vi "Voltage_overflow_checker.vi"() -> ()   [LabVIEW 2017]
uses:
  Globals/Meas_global.vi
panel:
  out "Over/Under string":string
  out "Extra Comments":string
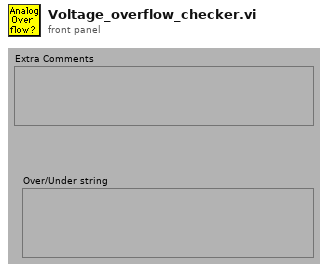
[diagram p1: front panel]
types:
  T1 = typedef "Analysis_info_cluster.ctl" = cluster{"Colour":u32, "Inst type":T2, "Inst name":string, "Symbol":string, "Code name":string, "Extra Info":string, "Inst Array":T3, "Extra Titles":string[], "Extra Values":string[], "U":dbl, "u^2":dbl, "u^3":dbl, "u^4":dbl, "Skew_u":dbl, "Kurt_u":dbl, "Sd Error in Mean":dbl, "% u'/U":dbl, "X":dbl, "Y":dbl, "Z":dbl, "Timescale integral Estimate":dbl, "Sd Error in Variance":dbl, "Calib File":path, "Calib Constants":dbl[], "Output Position":bool, "Full Stats":bool, "Av Sampling Rate":dbl, "Av No of Samples":dbl, "Total Meas Time (s)":dbl, "ADAM Ch Name":string, "Max value":dbl, "Min value":dbl, "Req Sample Rate Hz":dbl, "Sync Delay Time (s)":dbl, "Ch No":i16, "Device":string, "Use Latest Calib":bool, "Port":string, "Metadata Ch Names":string[], "Metadata Ch Values":string[]}
  T2 = typedef "Inst_type.ctl" = enum16{"Propeller anemometer", "Raw voltage", "Pressure Transducer", "Pitot-static tube", "Preston tube", "Hot wire", "Cross wire 1", "Cross wire 2", "Generic Linear", "Generic Polynomial", "Generic BackPoly", "Fast FID", "Thermocouple", "Cold wire", "Pulsed Wire", "LDA Vel", "LDA Tran time", "LDA Arr time", "Microphone"}
  T3 = typedef "Instrument_Array.ctl" = enum16{"PWA", "LDA", "Analogue"}
  T4 = typedef "Time_Trace_Cluster.ctl" = cluster{"Weighting":dbl[], "Time (s)":dbl[], "Voltage":dbl[], "Eng Values":dbl[]}
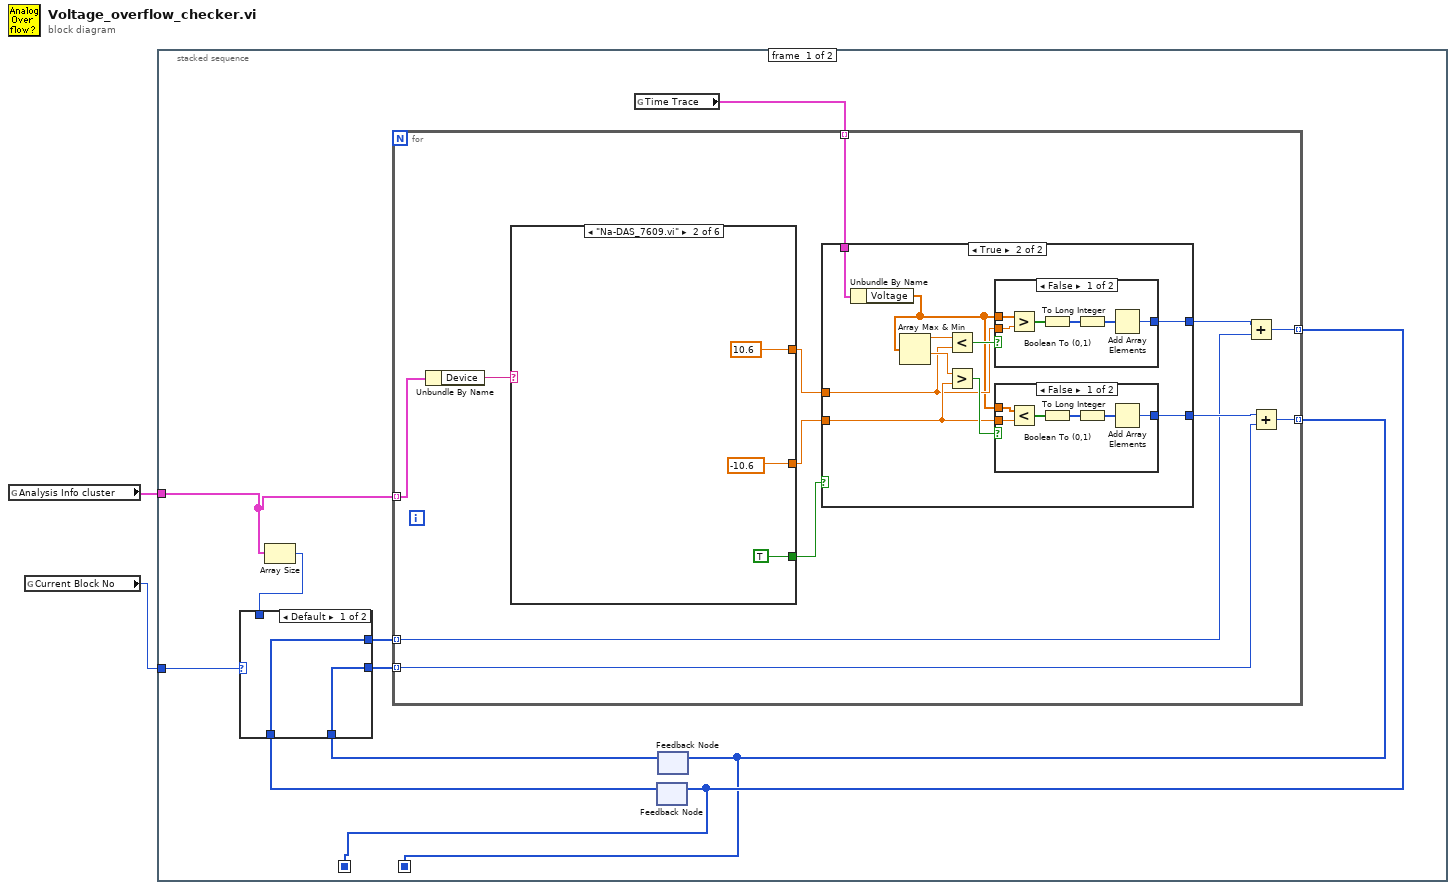
[diagram p0: block diagram]
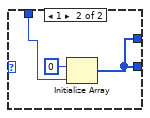
[diagram p2: hidden frame]
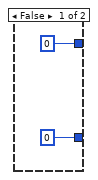
[diagram p3: hidden frame]
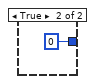
[diagram p4: hidden frame]
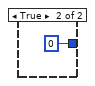
[diagram p5: hidden frame]
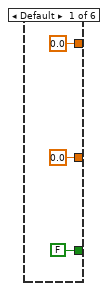
[diagram p6: hidden frame]
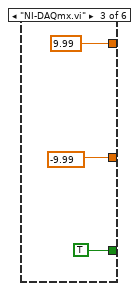
[diagram p7: hidden frame]
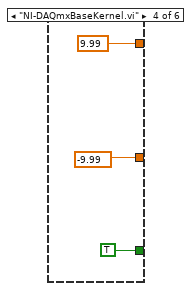
[diagram p8: hidden frame]
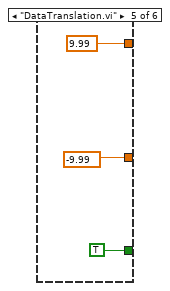
[diagram p9: hidden frame]
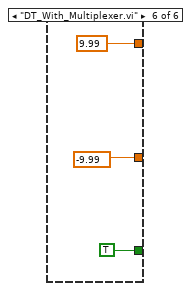
[diagram p10: hidden frame]
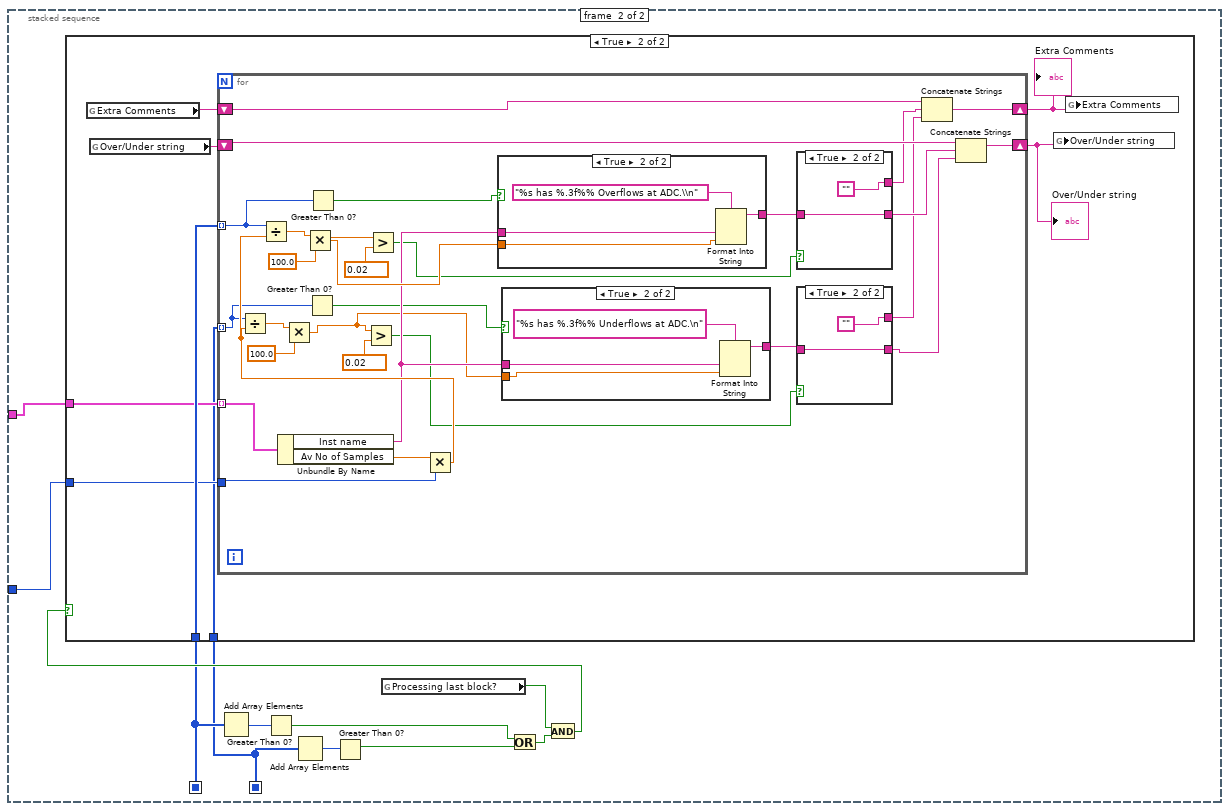
[diagram p11: hidden frame]
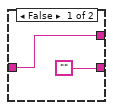
[diagram p13: hidden frame]
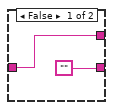
[diagram p14: hidden frame]
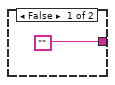
[diagram p15: hidden frame]
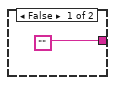
[diagram p16: hidden frame]
diagram:
  n1 = global read "Meas_global.vi" "Analysis Info cluster"() -> (w2:T1[])
  n2 = global read "Meas_global.vi" "Current Block No"() -> (w1:i32)
  n3 = stacked-sequence {
    seq-local: [w6 _] -> [_ w77]
    seq-local: [w5 _] -> [_ w74]
    tunnel: w2 -> [w3 w76]
    tunnel: w1 -> [w4 w75]
    frame #0 {
      n4 = Array Size(array=w3) -> (size(s)=w11:i32)
      n5 = global read "Meas_global.vi" "Time Trace"() -> (w12:T4[])
      n6 = feedback #1() -> (w9:i32[])  [unwired: 1 in]
      n7 = feedback #2() -> (w10:i32[])  [unwired: 1 in]
      n8 = case shown="Default" w4 {
        tunnel: w11 -> [_ w17]
        tunnel: [w14 w15] -> w8
        tunnel: w9 -> [w14 _]
        tunnel: [w13 w15] -> w7
        tunnel: w10 -> [w13 _]
        frame Default {
        }
        frame 1 {
          n9 = Initialize Array(0 ("element"), w17) -> (w15:i32[])
        }
      }
      n10 = for {
        tunnel: w12 -> [w26] mode=indexing
        tunnel: [w24] -> w6 mode=indexing
        tunnel: [w22] -> w5 mode=indexing
        tunnel: w8 -> [w21] mode=indexing
        tunnel: w7 -> [w20] mode=indexing
        tunnel: w3 -> [w18] mode=indexing
        n11 = Unbundle By Name(w18) -> ("Device"=w19:string)
        n12 = case shown="\"Na-DAS_7609.vi\"" w19 {
          tunnel: [FALSE TRUE TRUE TRUE TRUE TRUE] -> w29
          tunnel: [0.0 ("Min") -10.6 ("Min") -9.99 ("Min") -9.99 ("Min") -9.99 ("Min") -9.99 ("Min")] -> w28
          tunnel: [0.0 ("Max") 10.6 ("Max") 9.99 ("Max") 9.99 ("Max") 9.99 ("Max") 9.99 ("Max")] -> w27
          frame Default {
          }
          frame "Na-DAS_7609.vi" {
          }
          frame "NI-DAQmx.vi" {
          }
          frame "NI-DAQmxBaseKernel.vi" {
          }
          frame "DataTranslation.vi" {
          }
          frame "DT_With_Multiplexer.vi" {
          }
        }
        n13 = case shown="True" w29 {
          tunnel: [0 w38] -> w25
          tunnel: [0 w36] -> w23
          tunnel: w28 -> [_ w35]
          tunnel: w27 -> [_ w34]
          tunnel: w26 -> [_ w33]
          frame False {
          }
          frame True {
            n14 = Unbundle By Name(w33) -> ("Voltage"=w32:dbl[])
            n15 = Array Max & Min(array=w32) -> (max value=w41:dbl, min value=w40:dbl)  [unwired: 2 out]
            n16 = Less?(x=w41, y=w34) -> (x < y?=w39:bool)
            n17 = Greater?(x=w40, y=w35) -> (0:w37:bool)
            n18 = case shown="False" w39 {
              tunnel: w32 -> [w54 _]
              tunnel: w34 -> [w53 _]
              tunnel: [w50 0] -> w38
              frame False {
                n19 = Greater?(x=w54, y=w53) -> (0:w52:bool[])
                n20 = Boolean To (0,1)(Boolean=w52) -> (0, 1=w51:i16[])
                n21 = To Long Integer(number=w51) -> (32bit integer=w49:i32[])
                n22 = Add Array Elements(numeric array=w49) -> (sum=w50:i32)
              }
              frame True {
              }
            }
            n23 = case shown="False" w37 {
              tunnel: w32 -> [w47 _]
              tunnel: w35 -> [w46 _]
              tunnel: [w43 0] -> w36
              frame False {
                n24 = Less?(x=w47, y=w46) -> (x < y?=w45:bool[])
                n25 = Boolean To (0,1)(Boolean=w45) -> (0, 1=w44:i16[])
                n26 = To Long Integer(number=w44) -> (32bit integer=w42:i32[])
                n27 = Add Array Elements(numeric array=w42) -> (sum=w43:i32)
              }
              frame True {
              }
            }
          }
        }
        n28 = Add(x=w25, y=w21) -> (x+y=w24:i32)
        n29 = Add(x=w23, y=w20) -> (x+y=w22:i32)
      }
      n30 = feedback-in #1(w6) -> ()
      n31 = feedback-in #2(w5) -> ()
    }
    frame #1 {
      n32 = Add Array Elements(numeric array=w77) -> (sum=w83:i32)
      n33 = Greater Than 0?(x=w83) -> (x > 0?=w81:bool)
      n34 = Add Array Elements(numeric array=w74) -> (sum=w84:i32)
      n35 = Greater Than 0?(x=w84) -> (x > 0?=w82:bool)
      n36 = global read "Meas_global.vi" "Processing last block?"() -> (w79:bool)
      n37 = Or(x=w81, y=w82) -> (x .or. y?=w80:bool)
      n38 = And(x=w79, y=w80) -> (x .and. y?=w78:bool)
      n39 = case shown="True" w78 {
        tunnel: w77 -> [_ w92]
        tunnel: w76 -> [_ w91]
        tunnel: w75 -> [_ w90]
        tunnel: w74 -> [_ w89]
        frame False {
        }
        frame True {
          n40 = global read "Meas_global.vi" "Extra Comments"() -> (w85:string)
          n41 = global read "Meas_global.vi" "Over/Under string"() -> (w88:string)
          n42 = for {
            tunnel: w92 -> [w107] mode=indexing
            tunnel: w91 -> [w121] mode=indexing
            tunnel: w90 -> [w119]
            tunnel: w89 -> [w108] mode=indexing
            shift-right: [w101] -> w87
            shift-left: w88 -> [w102]
            shift-right: [w103] -> w86
            shift-left: w85 -> [w104]
            n43 = Unbundle By Name(w121) -> ("Inst name"=w110:string, "Av No of Samples"=w120:dbl)
            n44 = Greater Than 0?(x=w108) -> (x > 0?=w105:bool)
            n45 = Greater Than 0?(x=w107) -> (x > 0?=w106:bool)
            n46 = Multiply(x=w120, y=w119) -> (x*y=w114:dbl)
            n47 = Divide(x=w108, y=w114) -> (x/y=w115:dbl)
            n48 = Divide(x=w107, y=w114) -> (x/y=w118:dbl)
            n49 = Multiply(x=w115, y=100.0) -> (x*y=w109:dbl)
            n50 = Multiply(x=w118, y=100.0) -> (x*y=w112:dbl)
            n51 = Greater?(x=w109, y=0.02) -> (0:w95:bool)
            n52 = Greater?(x=w112, y=0.02) -> (0:w100:bool)
            n53 = case shown="True" w106 {
              tunnel: w112 -> [_ w138]
              tunnel: w110 -> [_ w137]
              tunnel: ["" w136] -> w98
              frame False {
              }
              frame True {
                n54 = Format Into String(format string="%s has %.3f%% Overflows at ADC.\\n" ("Format String"), w137, w138) -> (resulting string=w136:string)  [unwired: 2 in, 1 out]
              }
            }
            n55 = case shown="True" w105 {
              tunnel: w109 -> [_ w131]
              tunnel: w110 -> [_ w133]
              tunnel: ["" w132] -> w96
              frame False {
              }
              frame True {
                n56 = Format Into String(format string="%s has %.3f%% Underflows at ADC.\n" ("Format String"), w133, w131) -> (resulting string=w132:string)  [unwired: 2 in, 1 out]
              }
            }
            n57 = case shown="True" w100 {
              tunnel: ["" w129] -> w99
              tunnel: w98 -> [w126 w129]
              tunnel: [w126 ""] -> w97
              frame False {
              }
              frame True {
              }
            }
            n58 = case shown="True" w95 {
              tunnel: ["" w125] -> w94
              tunnel: w96 -> [w122 w125]
              tunnel: [w122 ""] -> w93
              frame False {
              }
              frame True {
              }
            }
            n59 = Concatenate Strings(w104, w97, w93) -> (w103:string)
            n60 = Concatenate Strings(w102, w99, w94) -> (w101:string)
          }
          "Extra Comments" <- w86
          "Over/Under string" <- w87
          n61 = global write "Meas_global.vi" "Over/Under string"(w87) -> ()
          n62 = global write "Meas_global.vi" "Extra Comments"(w86) -> ()
        }
      }
    }
  }
